vi "4-4  parrot.vi"() -> ()   [LabVIEW 2014]
doc: "This VI illustrates how to acquire a finite number of samples from a specified device. It requires the use of a microphone attached to the sound card. You can specify the number of samples to acquire, sample rate, number of channels and a bit rate per sample.\n------------------------------------\nAuther: Koji Ohashi\nCopyright (c) 2020 Japan LabVIEW Users Group, Volunteer members.\nThis VI is released under the MIT License.\nhttp://opensource.org/licenses/mit-license.php\n------------------------------------"
uses:
  <vilib>/sound2/lvsound2.llb/Sampling Mode.ctl
  <vilib>/sound2/lvsound2.llb/Sound Input Read (DBL).vi
  <vilib>/sound2/lvsound2.llb/Sound Output Write (DBL).vi
  <vilib>/sound2/lvsound2.llb/Sound Data Format.ctl
panel:
  in  "Recording Time (sec)":dbl=5.0
  in  "Sound Format":T1={"sample rate (S/s)"=22050.0, "number of channels"=2, "bits per sample"=16}
  in  "device ID (Out)":u32
  in  "Device ID":u32
  out "Sound Input":waveform(dbl)[](graph)
  out "Number of Samples/ch":i32=10000
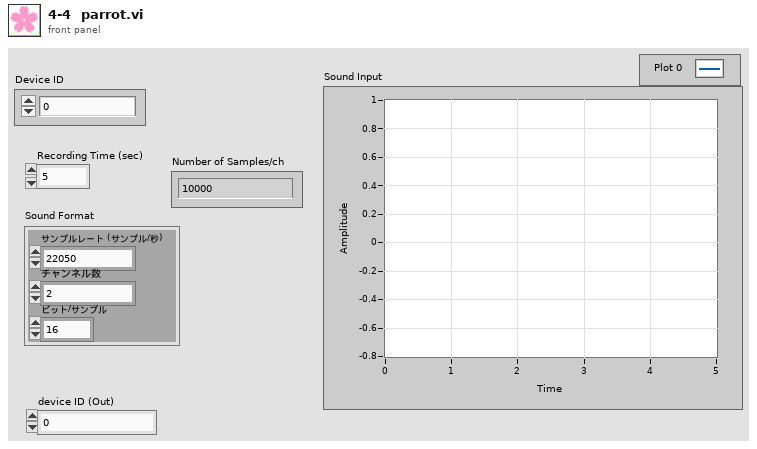
[diagram p1: front panel]
types:
  T1 = typedef "Sound Data Format.ctl" = cluster{"sample rate (S/s)":dbl, "number of channels":i32, "bits per sample":i32}
  T2 = typedef "Sampling Mode.ctl" = i32
  T3 = typedef "Sound Input Task ID.ctl" = u32
  T4 = typedef "Sound Output Task ID.ctl" = u32
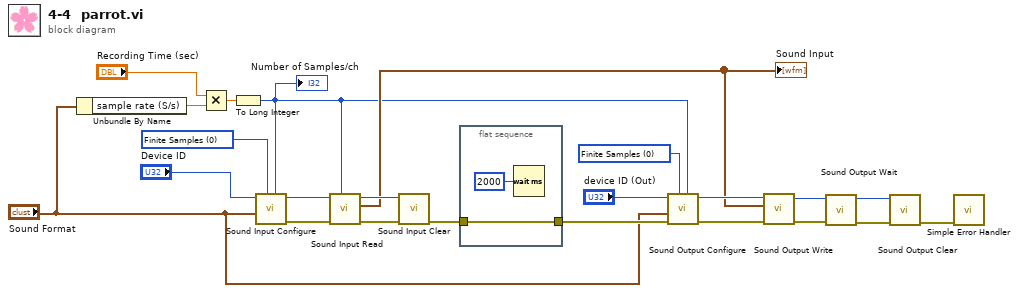
[diagram p0: block diagram]
diagram:
  w11 = T2 0 items=["Finite Samples", "Continuous Samples"] ("sample mode")
  w20 = T2 0 items=["Finite Samples", "Continuous Samples"] ("sample mode")
  n1 = Unbundle By Name("Sound Format") -> ("sample rate (S/s)"=w3:dbl)
  n2 = Multiply(x="Recording Time (sec)", y=w3) -> (x*y=w2:dbl)
  n3 = To Long Integer(number=w2) -> (32bit integer=w1:i32)
  "Number of Samples/ch" <- w1
  n4 = call <vilib>:"Sound Input Configure.vi"("number of samples/ch"=w1, "sample mode"=w20, "sound format"="Sound Format", "device ID"="Device ID") -> ("error out"=w23:errorcluster, "task ID"=w21:T3)  [unwired: 6 in]
  n5 = call-poly <vilib>:"Sound Input Read.vi"("number of samples/ch"=w1, "error in (no error)"=w23, "task ID"=w21) -> ("error out"=w18:errorcluster, "data"=w13:waveform(dbl)[], "task ID out"=w19:T3)  [unwired: 6 in]
  "Sound Input" <- w13
  n6 = call <vilib>:"Sound Input Clear.vi"("error in (no error)"=w18, "task ID"=w19) -> ("error out"=w17:errorcluster)  [unwired: 9 in]
  n7 = flat-sequence {
    tunnel: w17 -> [w25]
    tunnel: [w25] -> w16
    frame #0 {
      n8 = Wait (ms)(milliseconds to wait=u32 2000) -> ()  [unwired: 1 out]
    }
  }
  n9 = call <vilib>:"Sound Output Configure.vi"("number of samples/ch"=w1, "sample mode"=w11, "error in (no error)"=w16, "sound format"="Sound Format", "device ID"="device ID (Out)") -> ("error out"=w12:errorcluster, "task ID"=w14:T4)  [unwired: 5 in]
  n10 = call-poly <vilib>:"Sound Output Write.vi"("error in (no error)"=w12, "data"=w13, "task ID"=w14) -> ("error out"=w10:errorcluster, "task ID out"=w9:T4)  [unwired: 7 in]
  n11 = call <vilib>:"Sound Output Wait.vi"("error in (no error)"=w10, "task ID"=w9) -> ("error out"=w7:errorcluster, "task ID out"=w8:T4)  [unwired: 8 in]
  n12 = call <vilib>:"Sound Output Clear.vi"("error in (no error)"=w7, "task ID"=w8) -> ("error out"=w6:errorcluster)  [unwired: 9 in]
  n13 = call <vilib>:"Simple Error Handler.vi"("error in (no error)"=w6) -> ()  [unwired: 4 in, 5 out]
